vi "Test Cases - Cluster.vi"() -> ()   [LabVIEW 2017]
uses:
  db531f95-5889-428f-99e9-9bee3c65bca8.vi
  API-String-Arugments-Support/_Support/Data To API String Arguments.vi
  API-String-Arugments-Support/API String Arguments Support.lvlib
panel:
  out "String":string
  out "data":T1
  out "error 9":errorcluster
  out "Data 5":variant
  out "error 5":errorcluster
  out "Data 8":variant
  out "data 8":T2
  out "error 8":errorcluster
  out "Data 7":variant
  out "data 7":T2
  out "error 7":errorcluster
  out "Data 6":variant
  out "data 6":T2
  out "error 6":errorcluster
  out "error 1":errorcluster
  out "error 2":errorcluster
  out "error 3":errorcluster
  out "error 4":errorcluster
  out "Data 4":variant
  out "data 1":T2
  out "Data 1":variant
  out "Data 2":variant
  out "Data 3":variant
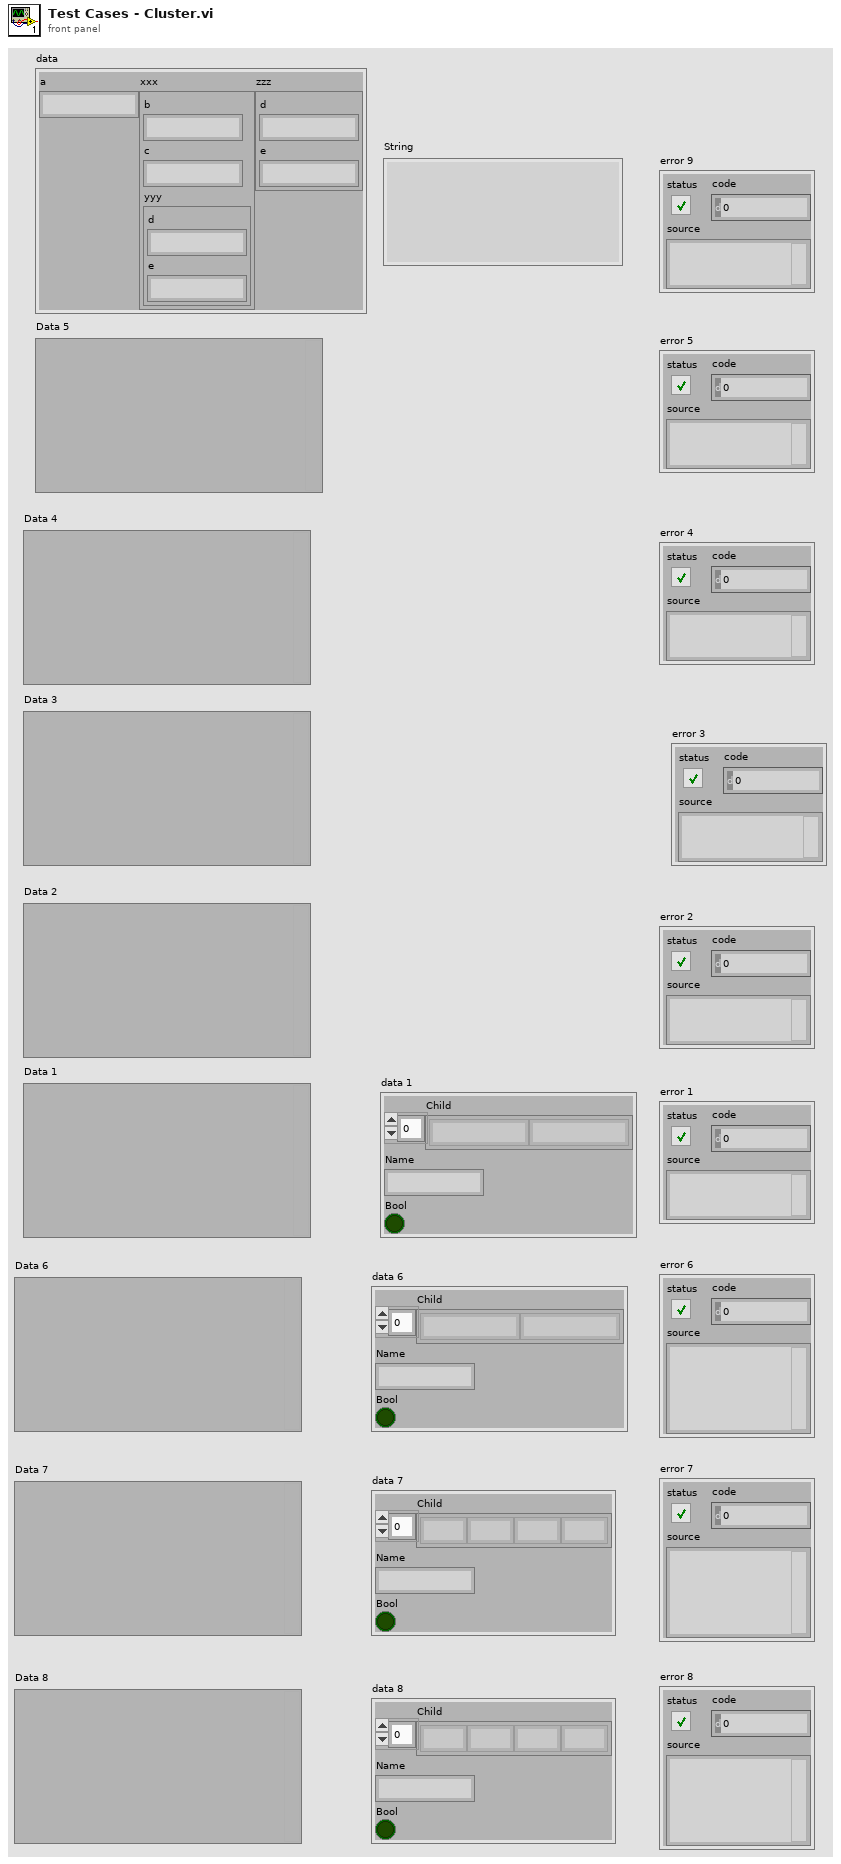
[diagram p1: front panel]
types:
  T1 = cluster{"a":string, "xxx":cluster{"b":string, "c":string, "yyy":cluster{"d":string, "e":string}}, "zzz":cluster{"d":string, "e":string}}
  T2 = cluster{"Child":string[], "Name":string, "Bool":bool}
  T3 = cluster{"Name":string, "Child":cluster{"Name":string}, "Bool":bool}
  T4 = cluster{"Child":cluster{"Name":string}, "Name":string, "Bool":bool}
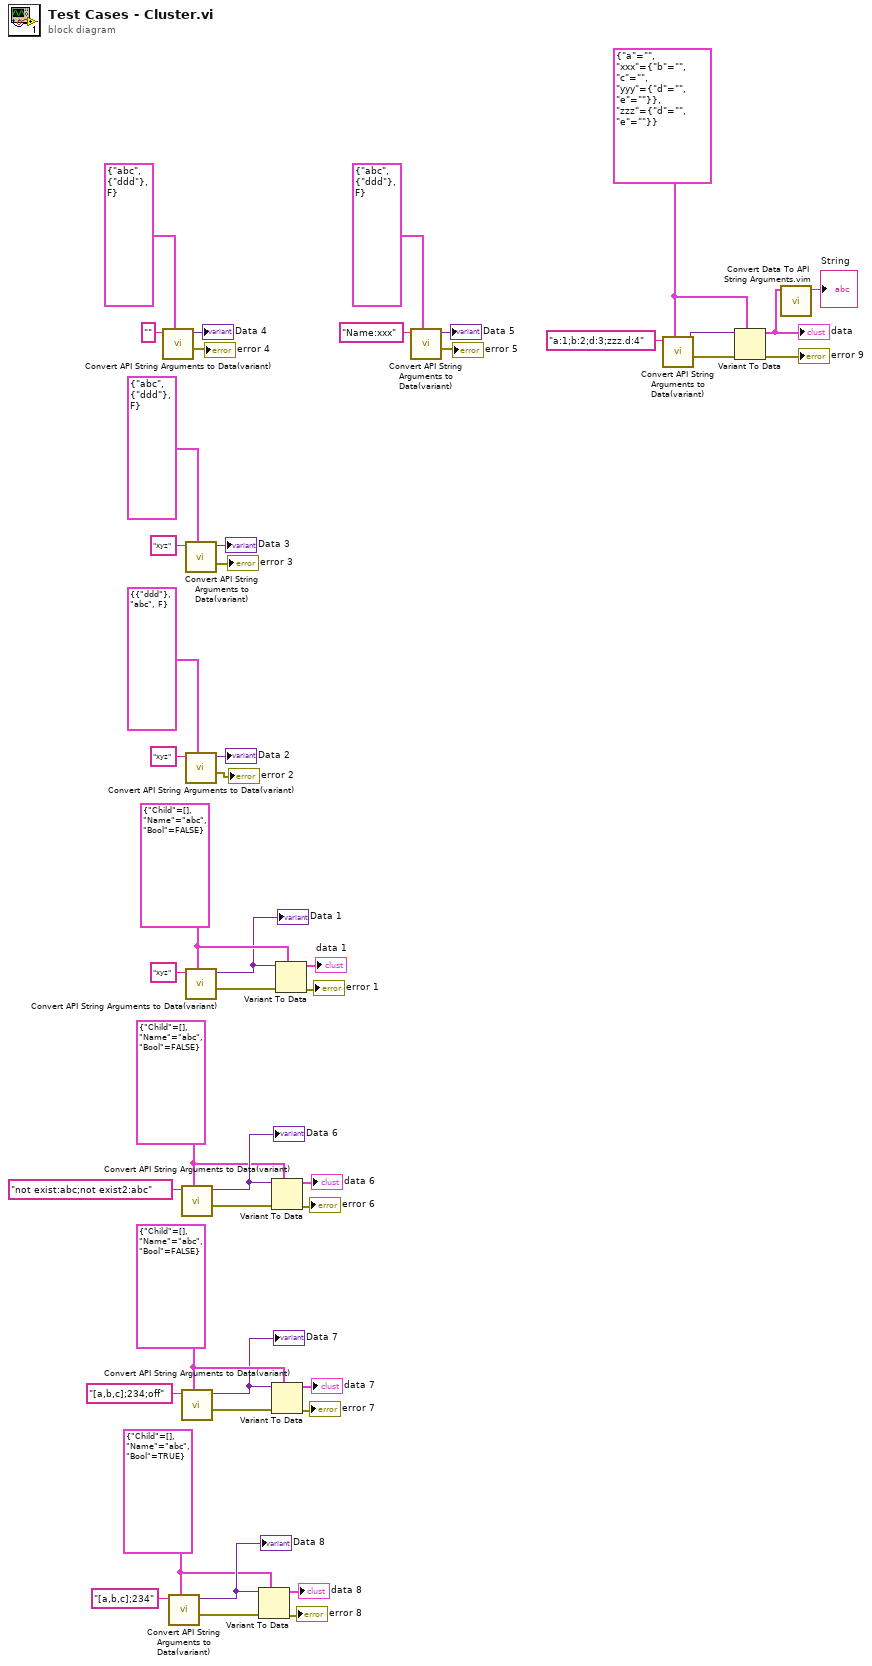
[diagram p0: block diagram]
diagram:
  w3 = T1 {"a"="", "xxx"={"b"="", "c"="", "yyy"={"d"="", "e"=""}}, "zzz"={"d"="", "e"=""}} ("Data 8")
  w14 = T2 {"Child"=[], "Name"="abc", "Bool"=TRUE} ("Data 8")
  w21 = T2 {"Child"=[], "Name"="abc", "Bool"=FALSE} ("Data 8")
  w26 = T2 {"Child"=[], "Name"="abc", "Bool"=FALSE} ("Data 8")
  w39 = T2 {"Child"=[], "Name"="abc", "Bool"=FALSE} ("Data 8")
  n1 = call "Convert API String Arguments to Data(variant).vi"("Type"=T3 {"Name"="abc", "Child"={"Name"="ddd"}, "Bool"=FALSE} ("Data 8"), "String"="") -> ("error"=→"error 4":errorcluster, "Data"=→"Data 4":variant)  [unwired: 8 in]
  n2 = call "Convert API String Arguments to Data(variant).vi"("Type"=w14, "String"="[a,b,c];234") -> ("error"=w13:errorcluster, "Data"=w15:variant)  [unwired: 8 in]
  "Data 8" <- w15
  n3 = call "Convert API String Arguments to Data(variant).vi"("Type"=w26, "String"="not exist:abc;not exist2:abc") -> ("error"=w25:errorcluster, "Data"=w27:variant)  [unwired: 8 in]
  "Data 6" <- w27
  n4 = call "Convert API String Arguments to Data(variant).vi"("Type"=w21, "String"="[a,b,c];234;off") -> ("error"=w22:errorcluster, "Data"=w20:variant)  [unwired: 8 in]
  "Data 7" <- w20
  n5 = call "Convert API String Arguments to Data(variant).vi"("Type"=T3 {"Name"="abc", "Child"={"Name"="ddd"}, "Bool"=FALSE} ("Data 8"), "String"="xyz") -> ("error"=→"error 3":errorcluster, "Data"=→"Data 3":variant)  [unwired: 8 in]
  n6 = call "Convert API String Arguments to Data(variant).vi"("Type"=T4 {"Child"={"Name"="ddd"}, "Name"="abc", "Bool"=FALSE} ("Data 8"), "String"="xyz") -> ("error"=→"error 2":errorcluster, "Data"=→"Data 2":variant)  [unwired: 8 in]
  n7 = call "Convert API String Arguments to Data(variant).vi"("Type"=w39, "String"="xyz") -> ("error"=w40:errorcluster, "Data"=w38:variant)  [unwired: 8 in]
  "Data 1" <- w38
  n8 = Variant To Data(error in=w13, type=w14, Variant=w15) -> (data=→"data 8":T2, error out=→"error 8":errorcluster)
  n9 = Variant To Data(error in=w25, type=w26, Variant=w27) -> (data=→"data 6":T2, error out=→"error 6":errorcluster)
  n10 = Variant To Data(error in=w22, type=w21, Variant=w20) -> (data=→"data 7":T2, error out=→"error 7":errorcluster)
  n11 = Variant To Data(error in=w40, type=w39, Variant=w38) -> (data=→"data 1":T2, error out=→"error 1":errorcluster)
  n12 = call "Convert API String Arguments to Data(variant).vi"("Type"=T3 {"Name"="abc", "Child"={"Name"="ddd"}, "Bool"=FALSE} ("Data 8"), "String"="Name:xxx") -> ("error"=→"error 5":errorcluster, "Data"=→"Data 5":variant)  [unwired: 8 in]
  n13 = call "Convert API String Arguments to Data(variant).vi"("Type"=w3, "String"="a:1;b:2;d:3;zzz.d:4") -> ("error"=w5:errorcluster, "Data"=w6:variant)  [unwired: 8 in]
  n14 = Variant To Data(error in=w5, type=w3, Variant=w6) -> (data=w2:T1, error out=→"error 9":errorcluster)
  "data" <- w2
  n15 = call "Convert Data To API String Arguments.vim"("data"=w2) -> ("String"=→"String":string)  [unwired: 7 in, 1 out]
